vi "Tosca-Execute Schedule Order Script (MATLAB).vi"(0 "Path":string, 11 "error in (no error)":errorcluster) -> (6 "result":string, 8 "order":i32[](array[numeric]), 15 "error out":errorcluster)   [LabVIEW 2020]
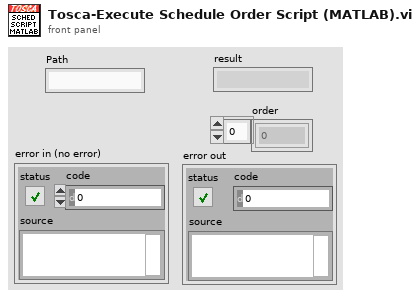
[diagram p1: front panel]
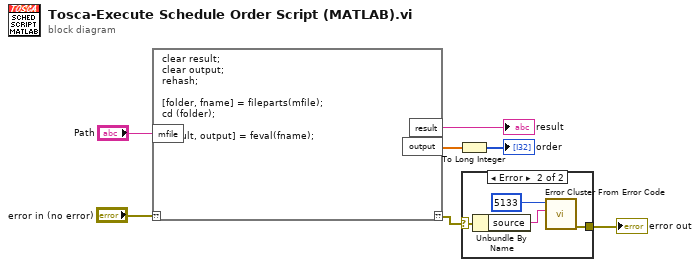
[diagram p0: block diagram]
diagram:
  n1 = script code="clear result;\nclear output;\nrehash;\n\n[folder, fname] = fileparts(mfile);\ncd (folder);\n\n[result, output] = feval(fname);"("??"="error in (no error)", "mfile"="Path") -> ("??"=w2:errorcluster, "result"=→"result":string, "output"=w7:dbl[])
  n2 = To Long Integer(number=w7) -> (32bit integer=→"order":i32[])
  n3 = case shown="Error" w2 {
    selector: w2 -> [w8 w10]
    tunnel: [w8 w11] -> w1
    frame No Error {
    }
    frame Error {
      n4 = Unbundle By Name(w10) -> ("source"=w9:string)
      n5 = call <vilib>:"Error Cluster From Error Code.vi"("error message (\"\")"=w9, "error code (0)"=5133) -> ("error out"=w11:errorcluster)  [unwired: 7 in]
    }
  }
  "error out" <- w1
